vi "Write Calibration.vi"(8 "error in (no error)":errorcluster, 10 "Calibration":dbl[unit], 11 "Analyze Parameter Calibration in":refnum<class "Analyze Parameter Calibration.lvclass">) -> (0 "error out":errorcluster, 3 "Analyze Parameter Calibration out":refnum<class "Analyze Parameter Calibration.lvclass">)   [LabVIEW 2014, in "Analyze Parameter Calibration.lvclass"]
uses:
  Analyze Parameter Calibration.lvclass
  Analyze Parameter Calibration.lvclass/Analyze Parameter Calibration.ctl
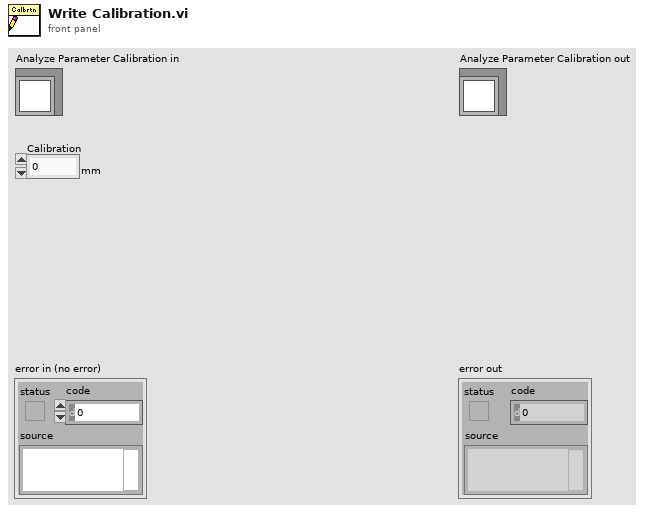
[diagram p1: front panel]
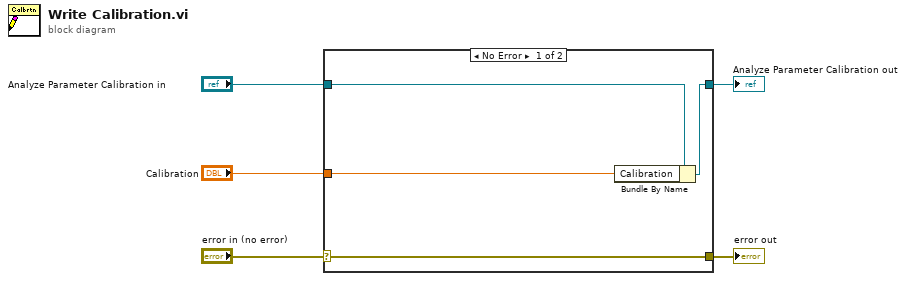
[diagram p0: block diagram]
diagram:
  n1 = case shown="No Error" "error in (no error)" {
    selector: "error in (no error)" -> [w9 w10]
    tunnel: [w9 w10] -> w4
    tunnel: [w7 w11] -> w2
    tunnel: "Analyze Parameter Calibration in" -> [w8 w11]
    tunnel: "Calibration" -> [w6 _]
    frame No Error {
      n2 = Bundle By Name(cluster=w8, "Calibration"=w6) -> (w7:refnum<class "Analyze Parameter Calibration.lvclass">)
    }
    frame Error {
    }
  }
  "error out" <- w4
  "Analyze Parameter Calibration out" <- w2
